vi "init_motion_commands.vi"(8 "error in (no error)":errorcluster caption="错误输入（无错误）", 10 "name":string, 11 "MotorSystem输入":refnum<class "MotorSystem.lvclass">) -> (0 "error out":errorcluster caption="错误输出", 3 "MotorSystem输出":refnum<class "MotorSystem.lvclass">)   [LabVIEW 2016, in "MotionControl_UFO_3DOF.lvlib" / "MotorSystem.lvclass"]
uses:
  <userlib>/MotionControl_UFO_3DOF/MotorSystem/MotorSystem.lvclass
  <userlib>/MotionControl_UFO_3DOF/MotorSystem/MotorSystem.lvclass/MotorSystem.ctl
  <userlib>/MotionControl_UFO_3DOF/OneMotion/OneMotion.lvclass
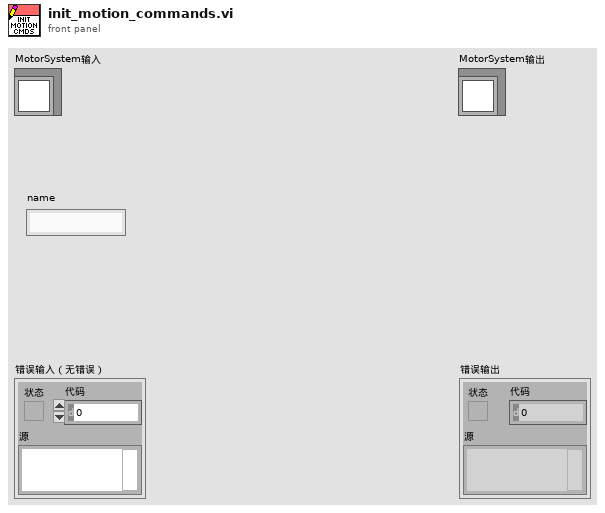
[diagram p1: front panel]
types:
  T1 = typedef "MotionControl_UFO_3DOF.lvlib/MotorSystem.lvclass/MotionCluster.ctl" = cluster{"OneMotion.lvclass":refnum<class "OneMotion.lvclass">, "connected?":bool, "default enabled?":bool, "enabled?":bool}
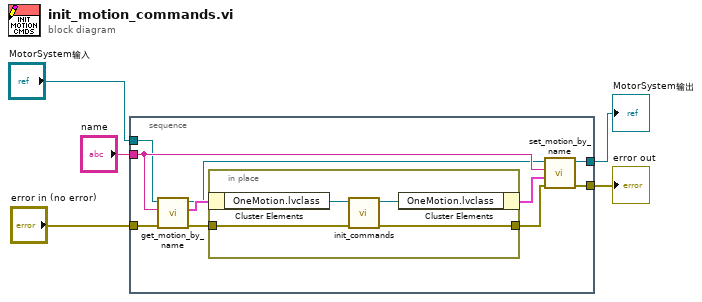
[diagram p0: block diagram]
diagram:
  n1 = stacked-sequence {
    tunnel: [w8] -> w5
    tunnel: [w12] -> w3
    tunnel: "MotorSystem输入" -> [w7]
    tunnel: "error in (no error)" -> [w9]
    tunnel: "name" -> [w13]
    frame #0 {
      n2 = call <userlib>:"get_motion_by_name.vi"("error in (no error)"=w9, "name"=w13, "MotorSystem in"=w7) -> ("error out"=w11:errorcluster, "motion cluster"=w15:T1, "MotorSystem out"=w6:refnum<class "MotorSystem.lvclass">)  [unwired: 6 in]
      n3 = in-place {
        in-place-border: w11 -> [w17]
        in-place-border: [w16] -> w10
        n4 = in-place-cluster #1(w15) -> ("OneMotion.lvclass"=w19:refnum<class "OneMotion.lvclass">)
        n5 = call-dynamic "init_commands.vi"("error in (no error)"=w17, "OneMotion 输入"=w19) -> ("error out"=w16:errorcluster, "OneMotion 输出"=w18:refnum<class "OneMotion.lvclass">)  [unwired: 8 in]
        n6 = in-place-cluster #1("OneMotion.lvclass"=w18) -> (w14:T1)
      }
      n7 = call <userlib>:"set_motion_by_name.vi"("error in (no error)"=w10, "簇"=w14, "name"=w13, "MotorSystem输入"=w6) -> ("error out"=w8:errorcluster, "MotorSystem输出"=w12:refnum<class "MotorSystem.lvclass">)  [unwired: 6 in]
    }
  }
  "error out" <- w5
  "MotorSystem输出" <- w3
